vi "FIR Filter with I.C..vi"   [LabVIEW 2010, in "NI_AALBase.lvlib"]
doc: "Filters the input sequence <B>X</B> using the direct-form FIR filter specified by <B>FIR Coefficients</B>. You can use this VI to process blocks of continuous data. Wire data to the <B>X</B> input to determine the polymorphic instance to use or manually select the instance."
uses:
  NI_AALBase.lvlib
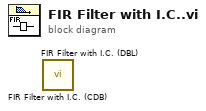
[diagram p0: block diagram]
diagram:
  n1 = call "FIR Filter with I.C. (CDB).vi"() -> ()  [unwired: 8 in, 3 out]
  n2 = call "FIR Filter with I.C. (DBL).vi"() -> ()  [unwired: 8 in, 3 out]
